vi "Set Error Status.vi"(10 "status (T)":bool=TRUE, 11 "error in":errorcluster) -> (3 "error out":errorcluster)   [LabVIEW 2027, in "Static Errors.lvlib"]
doc: "Sets the status of <b>error</b>."
uses:
  Static Errors.lvlib
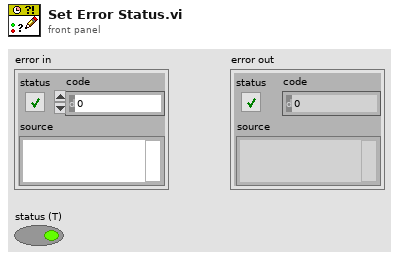
[diagram p1: front panel]
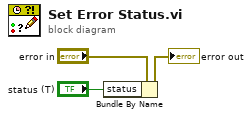
[diagram p0: block diagram]
diagram:
  n1 = Bundle By Name(cluster="error in", "status"="status (T)") -> (→"error out":errorcluster)
